vi "2_01.vi"() -> ()   [LabVIEW 2013]
uses:
  <vilib>/measure/NI_MABase.lvlib
  <vilib>/measure/NI_MAPro.lvlib
  <vilib>/measure/macond.llb/Continuous Waveform Convolution for 1 Chan.vi
panel:
  out "Waveform Graph":waveform(dbl)(graph)
  in  "Frecuencia":dbl
  in  "Nivel de Ruido":dbl
  in  "N":dbl
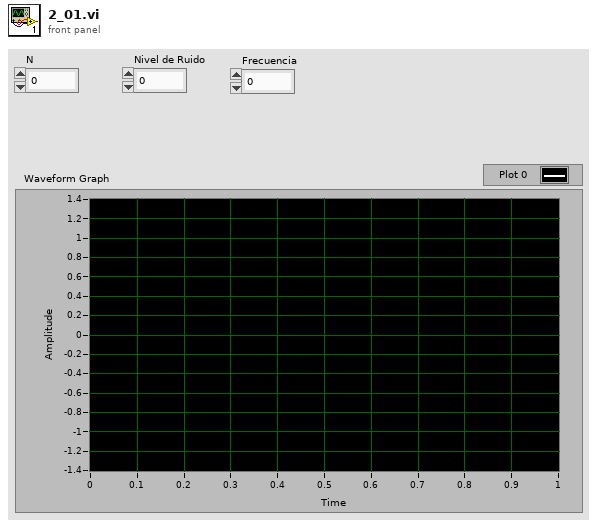
[diagram p1: front panel]
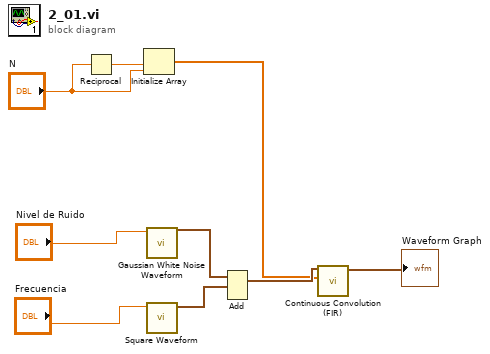
[diagram p0: block diagram]
diagram:
  n1 = Reciprocal(x="N") -> (1/x=w2:dbl)
  n2 = Initialize Array(w2, "N") -> (w3:dbl[])
  n3 = call <vilib>:"Gaussian White Noise Waveform.vi"("standard deviation"="Nivel de Ruido") -> ("signal out"=w7:waveform(dbl))  [unwired: 9 in, 1 out]
  n4 = call <vilib>:"Square Waveform.vi"("frequency"="Frecuencia") -> ("signal out"=w6:waveform(dbl))  [unwired: 9 in, 1 out]
  n5 = Add(1:w6, 2:w7) -> (0:w5:waveform(dbl))  [unwired: 1 in, 1 out]
  n6 = call-poly <vilib>:"Continuous Convolution (FIR).vi"("kernel"=w3, "signal in"=w5) -> ("signal out"=→"Waveform Graph":waveform(dbl))  [unwired: 8 in, 1 out]
